vi "Finish.vi"   [LabVIEW 2014]
doc: "This VI is called just before exiting. It is expected to close I/O refnum, save collected data, etc."
uses:
  TypeDefs/SRE Enum.ctl
types:
  T1 = typedef "SRE Enum.ctl" = enum16{"Start", "Run", "End"}
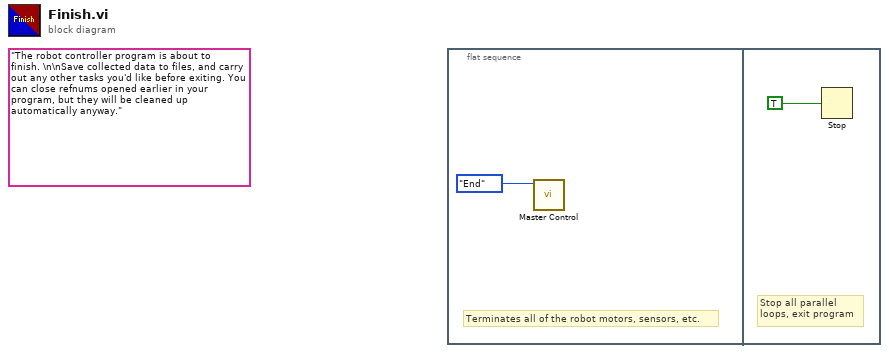
[diagram p0: block diagram]
diagram:
  (unwired) "The robot controller program is about to finish. \n\nSave collected data to files, and carry out any other tasks you'd like before exiting. You can close refnums opened earlier in your program, but they will be cleaned up automatically anyway."
  n1 = flat-sequence {
    frame #0 {
      # "Terminates all of the robot motors, sensors, etc."
      n2 = call "Master Control.vi"("Enum"=SRE_Enum."End") -> ()  [unwired: 11 in]
    }
    frame #1 {
      # "Stop all parallel\nloops, exit program"
      n3 = Stop(stop? (T)=TRUE ("Quit")) -> ()
    }
  }
